vi "time in Gamma - PID - V1.vi"(6 "nonzero temperature":dbl=300.0, 8 "adaptive sweep settings":T1={"time gap (min) "=0.0, "Bypass error dialog"=TRUE, "range factor"=1.05, "min gamma(kHz)"=0.005, "max step(Hz)"=1.05, "min step(Hz)"=0.005, "save freq units"=enum."Hz", "Zero synth"=FALSE, "time in Gamma --OK"=FALSE, "scan mode"=enum."predictive", "power control mode "=enum."power vs Temp", "time-in-gamma mode"=enum."same for all"}, 10 "sweep folder path":path, 11 "Fast sweep settings":T3={"Update rate (Hz)"=250.0, "Start F, Hz"=300000.0, "Stop F"=3500000.0, "Number of points"=23000, "Amplitude"=0.2, "Init&amplitude"=TRUE, "IF"=1000.0, "Time constant"=0.001} {"IF" format="%#_6p"; "Amplitude" min=0.0 max=2.5; "Number of points" format="%.0p"; "Stop F" format="%#_6p"; "Start F, Hz" format="%#_6p"; "Update rate (Hz)" format="%0.2f"}) -> (0 "adaptive sweep settings OUT":T1={"time gap (min) "=0.0, "Bypass error dialog"=TRUE, "range factor"=1.05, "min gamma(kHz)"=0.005, "max step(Hz)"=1.05, "min step(Hz)"=0.005, "save freq units"=enum."Hz", "Zero synth"=FALSE, "time in Gamma --OK"=FALSE, "scan mode"=enum."predictive", "power control mode "=enum."power vs Temp", "time-in-gamma mode"=enum."same for all"}, 1 "frequencies":dbl[](array[numeric]), 2 "temperatures":dbl[](array[numeric]), 3 "Fast sweep settings out":T3={"Update rate (Hz)"=250.0, "Start F, Hz"=200000.0, "Stop F"=1700000.0, "Number of points"=30000, "Amplitude"=2.1, "Init&amplitude"=TRUE, "IF"=1000.0, "Time constant"=0.1} {"IF" format="%#_6p"; "Amplitude" min=0.0 max=2.5; "Number of points" format="%.0p"; "Stop F" format="%#_6p"; "Start F, Hz" format="%#_6p"; "Update rate (Hz)" format="%0.2f"})   [LabVIEW 2012]
uses:
  RUS/Controls/Sweep settings.ctl
  adaptive sweep UI controls.ctl
  next chunk -- algorithm.ctl
  ctl -- name dispatcher -- action.ctl
  next chunk - read-write freq PID file - atomic actions .vi
  ctl -- name dispatcher.vi
  file -- 9w path.vi
  array -- find index - real.vi
  array -- interpolate -- i.vi
  Q -- check range -- i -- real.vi
  Q - not nan -- real.vi
  <vilib>/Utility/libraryn.llb/Check if File or Folder Exists.vi
  file -- read list of lines.vi
  parse -- find first line.vi
  parse -- get list of matches -- numbers.vi
panel:
  out "time in gamma":dbl
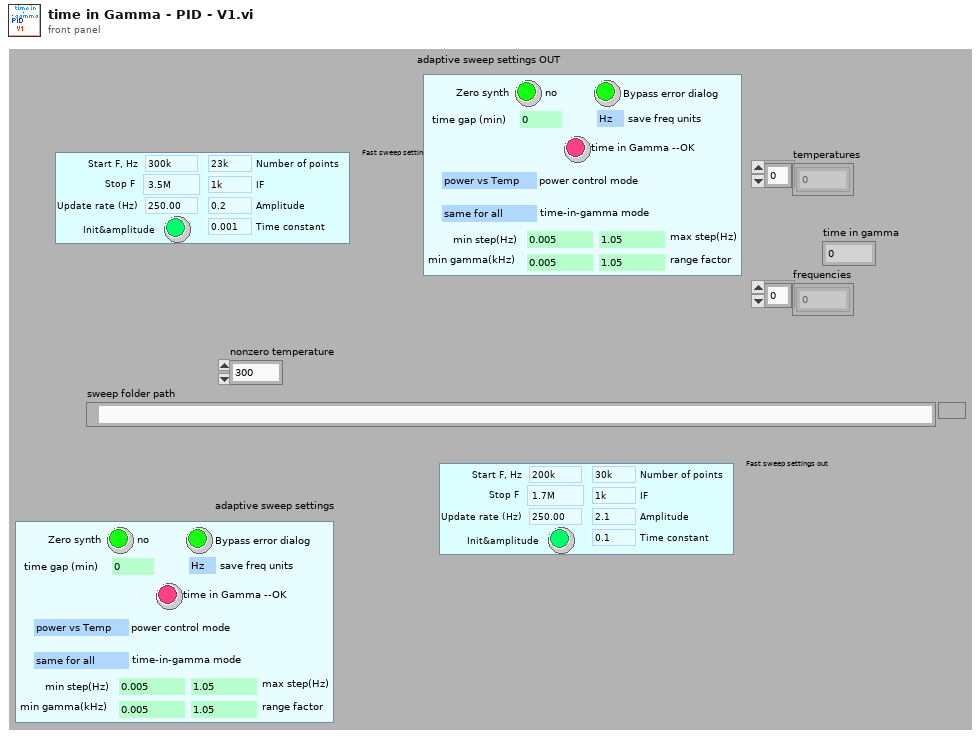
[diagram p1: front panel]
types:
  T1 = typedef "adaptive sweep UI controls.ctl" = cluster{"time gap (min) ":dbl, "Bypass error dialog":bool, "range factor":dbl, "min gamma(kHz)":dbl, "max step(Hz)":dbl, "min step(Hz)":dbl, "save freq units":enum16{"kHz", "Hz"}, "Zero synth":bool, "time in Gamma --OK":bool, "scan mode":T2, "power control mode ":enum16{"power vs Temp", "power vs Time", "none"}, "time-in-gamma mode":enum16{"same for all", "each one different", "uniform scan"}}
  T2 = typedef "next chunk -- algorithm.ctl" = enum16{"peak position is known", "uniform", "predictive"}
  T3 = typedef "Sweep settings.ctl" = cluster{"Update rate (Hz)":dbl, "Start F, Hz":dbl, "Stop F":dbl, "Number of points":i32, "Amplitude":dbl, "Init&amplitude":bool, "IF":dbl, "Time constant":dbl}
  T4 = enum16{"same for all", "each one different", "uniform scan"}
  T5 = typedef "ctl -- name dispatcher -- action.ctl" = enum16{"peak frequency", "peak frequency DUMP", "peak gamma DUMP", "peak gamma", "peak frequency TEST", "peak gamma TEST", "ultrasonic power", "time in gamma", "set temperature ", "set temperature timer", "peak default gamma", "last scan file", "peak freq gamma TEST", "peak NAMES", "errors", "P_I_D", "P", "I", "D", "power vs time", "power vs time TIMER", "void", "power log", "set temperature - SINE", "itc ltc log", "peak - time in gamma"}
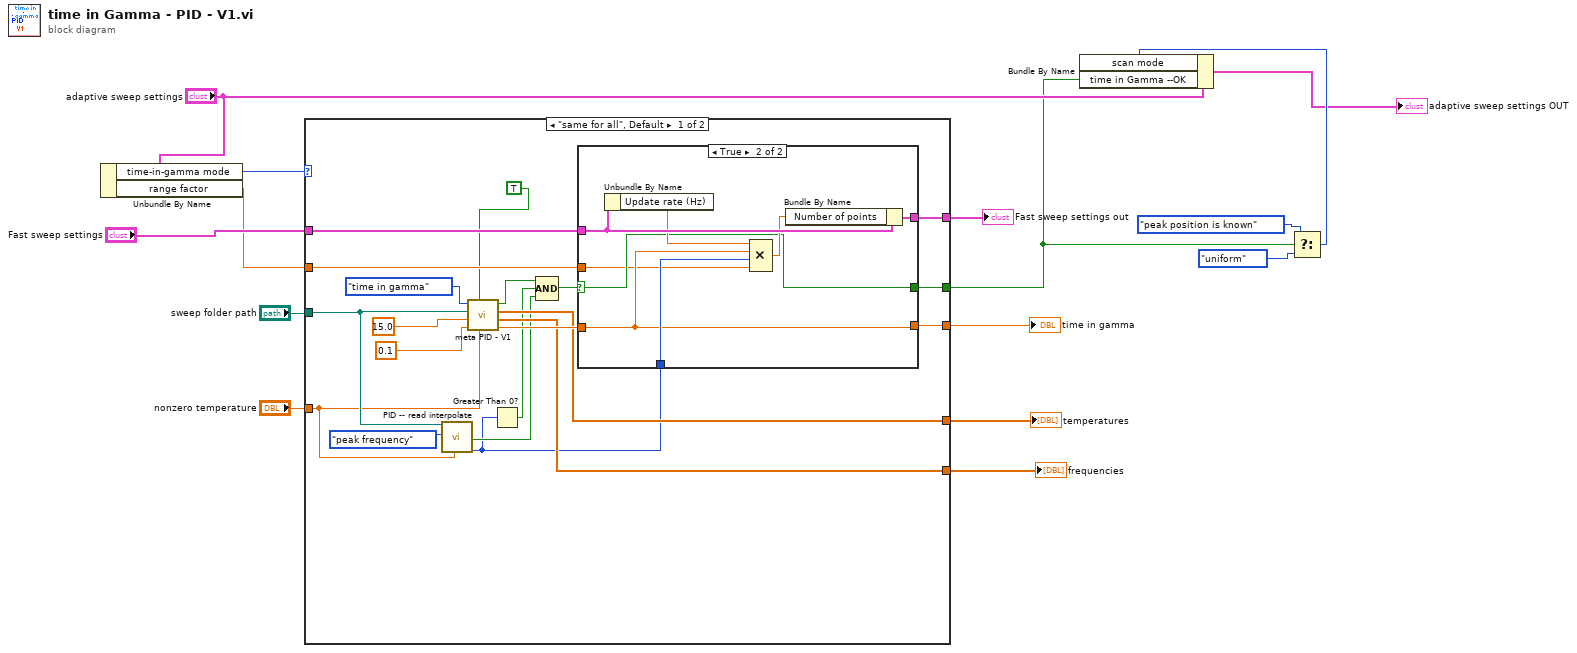
[diagram p0: block diagram]
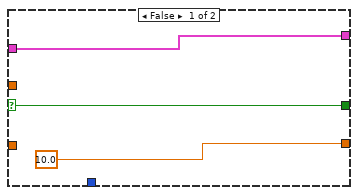
[diagram p2: hidden frame]
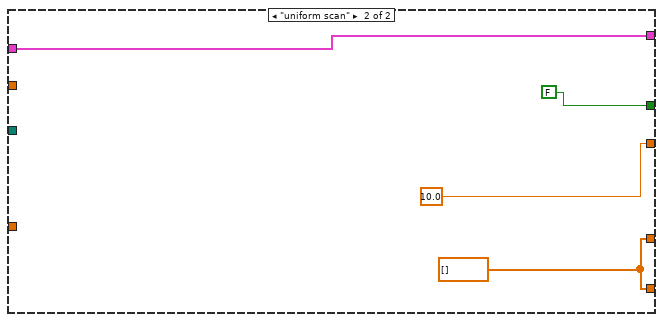
[diagram p3: hidden frame]
diagram:
  n1 = Unbundle By Name("adaptive sweep settings") -> ("time-in-gamma mode"=w6:T4, "range factor"=w1:dbl)
  n2 = case shown="\"same for all\", Default" w6 {
    tunnel: "Fast sweep settings" -> [w29 w50]
    tunnel: "sweep folder path" -> [w27 _]
    tunnel: "nonzero temperature" -> [w26 _]
    tunnel: [w28 w50] -> w12
    tunnel: [w35 10.0 ("upper")] -> w11
    tunnel: [w30 w48] -> w10
    tunnel: [w31 w48] -> w9
    tunnel: [w18 FALSE] -> w3
    tunnel: w1 -> [w17 _]
    frame "same for all", Default {
      n3 = call "PID -- read interpolate.vi"("sweep folder path"=w27, "ctl PID file IN"=ctl_--_name_dispatcher_--_action."peak frequency", "temperature"=w26) -> ("PID OK !"=w22:bool, "length out"=w21:i32)  [unwired: 11 in, 4 out]
      n4 = call "meta PID - V1.vi"("input parameter"=w26, "control?"=TRUE, "lower limit"=0.1 ("lower"), "upper limit"=15.0 ("upper"), "sweep folder path"=w27, "ctl name dispatch"=ctl_--_name_dispatcher_--_action."time in gamma") -> ("bezier output"=w32:dbl, "frequencies"=w31:dbl[], "temperatures"=w30:dbl[], "ok"=w24:bool)  [unwired: 2 in]
      n5 = Greater Than 0?(x=w21) -> (x > 0?=w25:bool)
      n6 = Compound Arithmetic op=AND(w24, w25, w22) -> (w23:bool)
      n7 = case shown="True" w23 {
        selector: w23 -> [w36 w40]
        tunnel: [w37 w46] -> w28
        tunnel: [10.0 ("upper") w44] -> w35
        tunnel: w32 -> [_ w44]
        tunnel: w29 -> [w37 w43]
        tunnel: w21 -> [_ w45]
        tunnel: [w36 w40] -> w18
        tunnel: w17 -> [_ w39]
        frame False {
        }
        frame True {
          n8 = Unbundle By Name(w43) -> ("Update rate (Hz)"=w42:dbl)
          n9 = Compound Arithmetic op=MULTIPLY(w42, w44, w45, w39) -> (w41:dbl)
          n10 = Bundle By Name(cluster=w43, "Number of points"=w41) -> (w46:T3)
        }
      }
    }
    frame "uniform scan" {
      w48 = dbl[] [] ("temperatures")
    }
  }
  "Fast sweep settings out" <- w12
  "time in gamma" <- w11
  "temperatures" <- w10
  "frequencies" <- w9
  n11 = Select(t=next_chunk_--_algorithm."peak position is known" ("next chunk algorithm"), s=w3, f=next_chunk_--_algorithm."uniform" ("next chunk algorithm")) -> (s? t:f=w4:T2)
  n12 = Bundle By Name(cluster="adaptive sweep settings", "scan mode"=w4, "time in Gamma --OK"=w3) -> (→"adaptive sweep settings OUT":T1)
